vi "Configure CAN Sample Point.vi"(8 "error in (no error)":errorcluster, 9 "Sample Point (0: 60)":i32(ring) items=["60", "62.5", "65", "67.5", "68", "70", "72.5", "75", "77.5", "80", "82.5", "85", "87.5"], 10 "CAN Channel (1: Channel 1)":i32(ring)=1 items=["Channel 1"=1, "Channel 2"=2, "Channel 3"=3, "Channel 4"=4], 11 "VISA resource name":refnum<visa-resource-name>) -> (0 "error out":errorcluster, 3 "VISA resource name out":refnum<visa-resource-name>)   [LabVIEW 2020, in "Agilent 90000 Series.lvlib"]
doc: "Sets the point during the bit time where the bit level is sampled to determine whether the bit is dominant or recessive. The sample point represents the percentage of time between the beginning of the bit time to the end of the bit time.\n\n<b>Note:</b>\nThis VI is new in firmware version 4.60."
uses:
  Agilent 90000 Series.lvlib
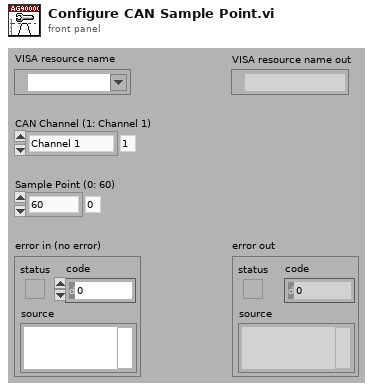
[diagram p1: front panel]
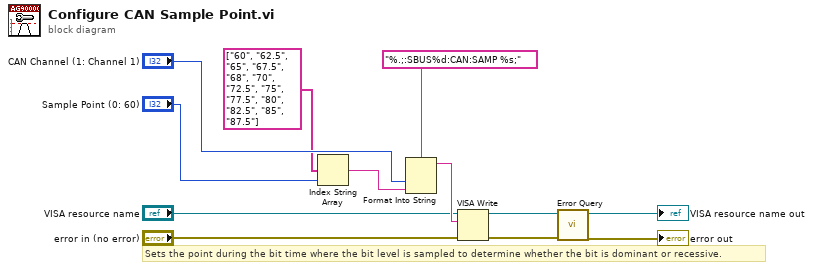
[diagram p0: block diagram]
diagram:
  # "Sets the point during the bit time where the bit level is sampled to determine whether the bit is dominant or recessive."
  n1 = Index String Array(1:"Sample Point (0: 60)", 2:string[] ["60", "62.5", "65", "67.5", "68", "70", "72.5", "75", "77.5", "80", "82.5", "85", "87.5"] ("string array")) -> (0:w3:string)  [unwired: 1 in]
  n2 = Format Into String(format string="%.;:SBUS%d:CAN:SAMP %s;", "CAN Channel (1: Channel 1)", w3) -> (resulting string=w11:string)  [unwired: 2 in, 1 out]
  n3 = VISA Write(VISA resource name="VISA resource name", write buffer=w11, error in (no error)="error in (no error)") -> (VISA resource name out=w8:refnum<visa-resource-name>, error out=w7:errorcluster)  [unwired: 1 out]
  n4 = call "Error Query.vi"("error in (no error)"=w7, "VISA resource name"=w8) -> ("error out"=→"error out":errorcluster, "VISA resource name out"=→"VISA resource name out":refnum<visa-resource-name>)  [unwired: 6 in, 2 out]
